vi "read-mxp.vi"() -> ()   [LabVIEW 2018]
uses:
  bno055.ctl
  <vilib>/Rock Robotics/WPI/SerialPort/WPI_SerialPort.ctl
  <vilib>/Rock Robotics/SystemInterfaces/AI/FPGA_AIChannel.ctl
panel:
  out "Bytes at Port":u32
  out "Array":dbl[](array[numeric])
  out "BNO055":T1
  in  "stop":bool
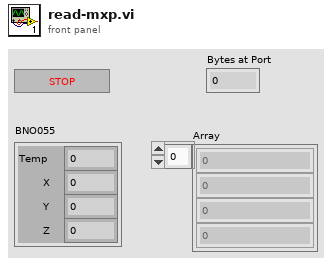
[diagram p1: front panel]
types:
  T1 = typedef "bno055.ctl" = cluster{"Temp":dbl, "X":dbl, "Y":dbl, "Z":dbl}
  T2 = typedef "FPGA_AIChannel.ctl" = enum8{"AI 0", "AI 1", "AI 2", "AI 3", "AI MXP 0", "AI MXP 1", "AI MXP 2", "AI MXP 3", "Invalid"}
  T3 = typedef "WPI_SerialPort.ctl" = enum16{"Onboard RS-232", "MXP TTL", "USB 1", "USB 2"}
  T4 = typedef "WPI_SerialPortRef.ctl" = cluster{"DevStatus":errorcluster, "Serial Port Name":refnum<visa-resource-name>}
  T5 = typedef "WPI_AnalogChannelDevRef.ctl" = cluster{"DevStatus":errorcluster, "Analog Channel":T2}
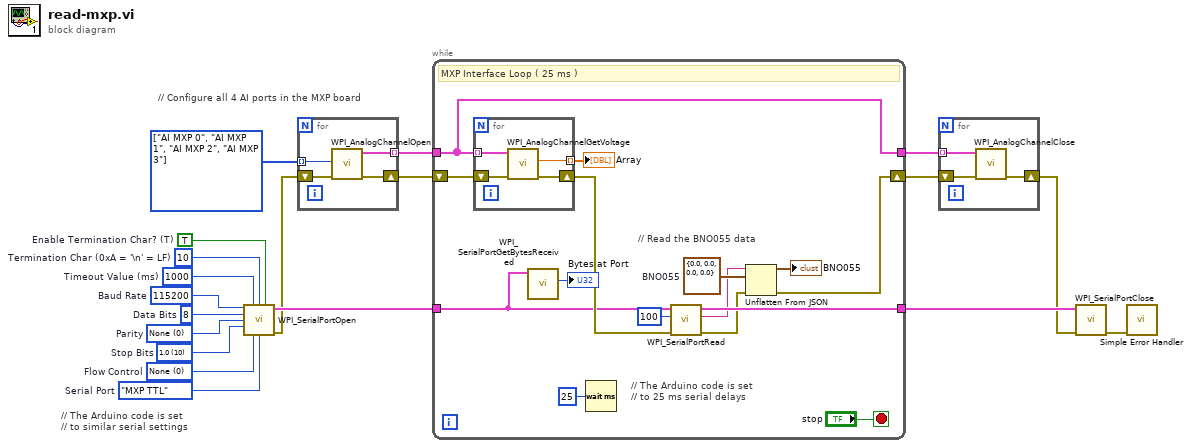
[diagram p0: block diagram]
diagram:
  w6 = T2[] [enum."AI MXP 0", enum."AI MXP 1", enum."AI MXP 2", enum."AI MXP 3"] items=["AI 0", "AI 1", "AI 2", "AI 3", "AI MXP 0", "AI MXP 1", "AI MXP 2", "AI MXP 3", "Invalid"]
  w11 = WPI_SerialPort."MXP TTL"  # Serial Port
  w12 = u16 0 items=["None", "XON/XOFF", "RTS/CTS", "XON/XOFF & RTS/CTS", "DTR/DSR", "XON/XOFF & DTR/DSR"]  # Flow Control
  w13 = u16 10 items=["1.0"=10, "1.5"=15, "2.0"=20]  # Stop Bits
  w14 = u16 0 items=["None", "Odd", "Even", "Mark", "Space"]  # Parity
  w10 = u16 8  # Data Bits
  w15 = u32 115200  # Baud Rate
  w16 = u32 1000  # Timeout Value (ms)
  w17 = u8 10  # Termination Char (0xA = '\n' = LF)
  w18 = TRUE  # Enable Termination Char? (T)
  # "// Configure all 4 AI ports in the MXP board"
  # "// The Arduino code is set \n// to similar serial settings"
  n1 = call <vilib>:"WPI_SerialPortOpen.vi"("Baud Rate"=w15, "Timeout Value (ms)"=w16, "Termination Char (0xA = '\\n' = LF)"=w17, "Enable Termination Char? (T)"=w18, "Data Bits"=w10, "Parity"=w14, "Stop Bits"=w13, "Flow Control"=w12, "Serial Port"=w11) -> ("SerialPortRef"=w9:T4, "error out"=w7:errorcluster)  [unwired: 5 in]
  n2 = for {
    tunnel: w6 -> [w22] mode=indexing
    shift-right: [w21] -> w1
    shift-left: w7 -> [w23]
    tunnel: [w20] -> w3 mode=indexing
    n3 = call <vilib>:"WPI_AnalogChannelOpen.vi"("error in (no error)"=w23, "Analog Channel"=w22) -> ("error out"=w21:errorcluster, "AIDeviceRef"=w20:T5)  [unwired: 8 in]
  }
  n4 = while "MXP Interface Loop" {
    shift-right: [w28] -> w5
    shift-left: w1 -> [w30]
    tunnel: w9 -> [w25]
    tunnel: [w38] -> w8
    tunnel: w3 -> [w26]
    tunnel: [w26] -> w2
    stop <- "stop" stop-if-true
    w34 = T1 {"Temp"=0.0, "X"=0.0, "Y"=0.0, "Z"=0.0}  # BNO055
    # "// Read the BNO055 data"
    # "// The Arduino code is set \n// to 25 ms serial delays"
    # "MXP Interface Loop ( 25 ms )"
    n5 = for {
      shift-right: [w40] -> w29
      shift-left: w30 -> [w41]
      tunnel: w26 -> [w42] mode=indexing
      tunnel: [w39] -> w27 mode=indexing
      n6 = call <vilib>:"WPI_AnalogChannelGetVoltage.vi"("error in (no error)"=w41, "AIDeviceRef"=w42) -> ("error out"=w40:errorcluster, "Voltage"=w39:dbl)  [unwired: 7 in, 1 out]
    }
    "Array" <- w27
    n7 = call <vilib>:"WPI_SerialPortGetBytesReceived.vi"("SerialPortRef"=w25) -> ("Bytes at Port"=→"Bytes at Port":u32)  [unwired: 8 in, 2 out]
    n8 = Wait (ms)(milliseconds to wait=u32 25) -> ()  [unwired: 1 out]
    n9 = call <vilib>:"WPI_SerialPortRead.vi"("error in (no error)"=w29, "Num Bytes to Read"=u32 100, "SerialPortRef"=w25) -> ("error out"=w33:errorcluster, "Buffer"=w31:string, "SerialPortRef"=w38:T4)  [unwired: 6 in]
    n10 = Unflatten From JSON(JSON string=w31, type and defaults=w34, error in (no error)=w33) -> (value=→"BNO055":T1, error out=w28:errorcluster)  [unwired: 4 in]
  }
  n11 = for {
    shift-right: [w44] -> w4
    shift-left: w5 -> [w45]
    tunnel: w2 -> [w43] mode=indexing
    n12 = call <vilib>:"WPI_AnalogChannelClose.vi"("error in (no error)"=w45, "AIDeviceRef"=w43) -> ("error out"=w44:errorcluster)  [unwired: 9 in]
  }
  n13 = call <vilib>:"WPI_SerialPortClose.vi"("error in (no error)"=w4, "SerialPortRef"=w8) -> ("error out"=w19:errorcluster)  [unwired: 9 in]
  n14 = call <vilib>:"Simple Error Handler.vi"("error in (no error)"=w19) -> ()  [unwired: 4 in, 5 out]
